vi "Get Config File Path.vi"(8 "error in (no error)":errorcluster) -> (0 "error out":errorcluster, 3 "Config Directory":path)   [LabVIEW 2020, in "Paths.lvlib"]
doc: "Generates the default configuration path. \nWhen called from the development environement, the default config path is the /Config relative to the project path.\nWhen called from a built exe the default config path is at C:\\Users\\<username>\\AppData\\Local\\<CompanyName>\\<ProductName> where company name and product name are the ones configured in the build specification.\nOn Linux the default config directory is \\home\\lvuser\\natinst\\bin\\config."
uses:
  Paths.lvlib
  <vilib>/Utility/sysdir.llb/System Directory Type.ctl
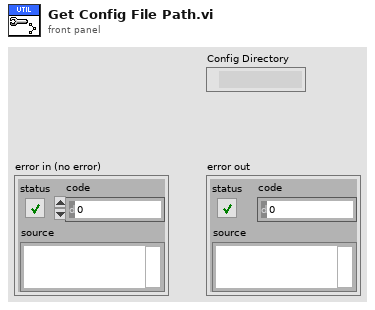
[diagram p1: front panel]
types:
  T1 = typedef "System Directory Type.ctl" = i32
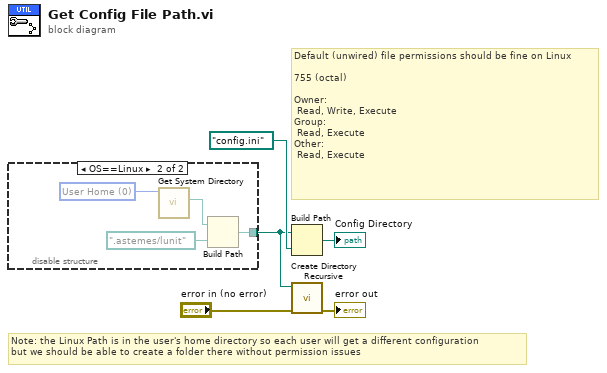
[diagram p0: block diagram]
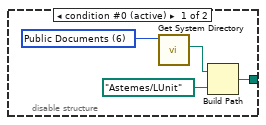
[diagram p2: hidden frame]
diagram:
  # "Note: the Linux Path is in the user's home directory so each user will get a different configuration \nbut we should be able to create a folder there without permission issues"
  # "Default (unwired) file permissions should be fine on Linux\n\n755 (octal) \n\nOwner:\n Read, Write, Execute\nGroup:\n Read, Execute\nOther:\n Read, Execute"
  n1 = disable-structure shown="OS==Linux" {
    disable-tunnel: [w9 w10] -> w1
    frame condition #0 (active) {
      w8 = T1 6 items=["User Home"=0, "User Desktop"=1, "User Documents"=2, "User Application Data"=3, "User Preferences"=4, "User Temporary"=5, "Public Documents"=6, "Public Application Data"=7, "Public Preferences"=8, "Public Cache"=13, "System Core Libraries"=9, "System Installed Libraries"=10, "Application Files"=11, "Boot Volume Root"=12] ("system directory type")
      n2 = call <vilib>:"Get System Directory.vi"("system directory type"=w8) -> ("system directory"=w6:path)  [unwired: 10 in]
      n3 = Build Path(base path=w6, name or relative path=path "Astemes/LUnit") -> (appended path=w9:path)
    }
    frame condition #1 {
      w13 = T1 0 items=["User Home"=0, "User Desktop"=1, "User Documents"=2, "User Application Data"=3, "User Preferences"=4, "User Temporary"=5, "Public Documents"=6, "Public Application Data"=7, "Public Preferences"=8, "Public Cache"=13, "System Core Libraries"=9, "System Installed Libraries"=10, "Application Files"=11, "Boot Volume Root"=12] ("system directory type")
      n4 = call <vilib>:"Get System Directory.vi"("system directory type"=w13) -> ("system directory"=w11:path)  [unwired: 10 in]
      n5 = Build Path(base path=w11, name or relative path=path ".astemes/lunit") -> (appended path=w10:path)
    }
  }
  n6 = Build Path(base path=w1, name or relative path=path "config.ini") -> (appended path=→"Config Directory":path)
  n7 = call <vilib>:"Create Directory Recursive.vi"("error in (no error)"="error in (no error)", "directory"=w1) -> ("error out"=→"error out":errorcluster)  [unwired: 3 in, 2 out]
